vi "write_channel.vi"(7 "error in (no error)":errorcluster, 9 "Channel":T1={"State"=FALSE, "Channel"=1, "Delay"=0.0, "Sync"="T0", "Width"=0.0, "Mode"="TTL", "Polarity"="NORM", "Amplitude"=0.0} {"Amplitude" format="%#.9g"; "Width" format="%#.9g"; "Delay" format="%.9f"; "Channel" items=["CHA"=1, "CHB"=2, "CHC"=3, "CHD"=4, "CHE"=5, "CHF"=6, "CHG"=7, "CHH"=8]}, 10 "VISA resource name":refnum<visa-resource-name>) -> (0 "error out":errorcluster, 3 "VISA resource name out":refnum<visa-resource-name>)   [LabVIEW 2012]
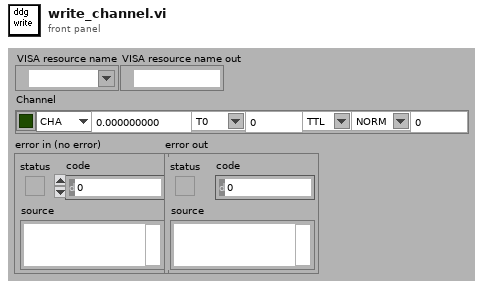
[diagram p1: front panel]
types:
  T1 = cluster{"State":bool, "Channel":u16, "Delay":dbl, "Sync":string, "Width":dbl, "Mode":string, "Polarity":string, "Amplitude":dbl}
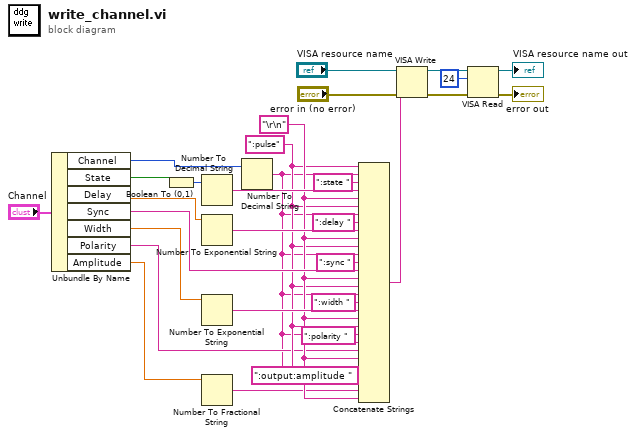
[diagram p0: block diagram]
diagram:
  w8 = "\r\n" ("string")
  w7 = ":pulse" ("string")
  n1 = Unbundle By Name("Channel") -> ("Channel"=w23:u16, "State"=w22:bool, "Delay"=w20:dbl, "Sync"=w16:string, "Width"=w19:dbl, "Polarity"=w5:string, "Amplitude"=w4:dbl)
  n2 = Boolean To (0,1)(Boolean=w22) -> (0, 1=w21:i16)
  n3 = Number To Decimal String(number=w21) -> (decimal integer string=w18:string)  [unwired: 1 in]
  n4 = Number To Exponential String(number=w20) -> (E-format string=w17:string)  [unwired: 3 in]
  n5 = Number To Exponential String(number=w19) -> (E-format string=w15:string)  [unwired: 3 in]
  n6 = Number To Fractional String(number=w4) -> (F-format string=w1:string)  [unwired: 3 in]
  n7 = Number To Decimal String(number=w23) -> (decimal integer string=w3:string)  [unwired: 1 in]
  n8 = Concatenate Strings(w7, w3, ":state " ("string"), w18, w8, w7, w3, ":delay " ("string"), w17, w8, w7, w3, ":sync " ("string"), w16, w8, w7, w3, ":width " ("string"), w15, w8, w7, w3, ":polarity " ("string"), w5, w8, w7, w3, ":output:amplitude " ("string"), w1, w8) -> (w26:string)
  n9 = VISA Write(VISA resource name="VISA resource name", write buffer=w26, error in (no error)="error in (no error)") -> (VISA resource name out=w13:refnum<visa-resource-name>, error out=w14:errorcluster)  [unwired: 1 out]
  n10 = VISA Read(VISA resource name=w13, byte count=u32 24, error in (no error)=w14) -> (VISA resource name out=→"VISA resource name out":refnum<visa-resource-name>, error out=→"error out":errorcluster)  [unwired: 2 out]
